vi "STAGE+mono+counter_edit5.vi"() -> ()   [LabVIEW 2017]
panel:
  out "Spectrum 2":waveform(dbl)(graph)
  out "XY Graph":cluster{"Y":dbl[], "Y":dbl[]}[](graph)
  in  "Integrating time, 10^-7 sec":dbl=10000000.0
  out "Timeout 2":bool
  in  "scan from":i32=2600
  in  "scan to":i32=4000
  in  "?":bool
  in  "Exit Labview":bool
  in  "step size":dbl=10.0 min=0.0
  in  "?":bool
  out "Spectrum":waveform(dbl)(graph)
  out "Counts":i32
  in  "value (0)":dbl=-9.0
  out "Current WL Wavelength  2":u16 caption="Current Wavelength"
  out "Grt# 2":u8=1 min=1 max=3 step=1
  out "Blaze (nm)":u32=300
  out "Groove/mm":u32=1200
  in  "?":bool
  in  "Channel B Input":u16(ring)=2 items=["Input 1"=1, "Input 2"=2]
  in  "Trigger mode":u16(ring) items=["10 MHz"=0, "Input 2"=2, "Input T"=3]
  out "Current WL Wavelength":u16 caption="Current Wavelength"
  in  "Integrating time, 10^-7 sec":dbl=10000000.0
  in  "gate A mode (CW:0)":i16(slide) scale=0.0..2.0 scale format="%.2f"
  in  "Channel A Input":u16(ring)=1 items=["10 MHz", "Input 1"]
  in  "Time between measurements\n at one point (s)/Dwell Time":dbl=0.002 min=0.002 max=60.0 step=0.001
  in  "Number of Measurements\n to take at one point/ Number of Periods":u16=1 min=1 max=2000 step=1
  in  "Count Mode":u16(ring) items=["A,B for Preset T", "A-B for Preset T", "A+B for Preset T", "A for Preset B"]
  in  "GPIB address":string="23"
  out "Timeout":bool
  out "Serial":u32=12345
  out "Grt#":u8=1 min=1 max=3 step=1
  out "Blaze (nm)":u32=300
  out "Groove/mm":u32=1200
  out "time delay":u32=450000 min=1
  out "Mono port":T1(ring)
  in  "Get position":bool
  out "Position status":dbl format="%.3f"
  in  "Target position":dbl format="%.3f"
  in  "Move":bool
  in  "Motor OFF":bool
  in  "Motor ON":bool
  in  "Step Size [um]":i32=10
  in  "Axis":i32=1
  in  "Rep Rate [Hz]":dbl=500.0
  out "Shots":dbl
  in  "Averaging Time [s]":dbl=0.1
  out "Current Point":i32
  out "Slide":i32(slide) scale=0.0..100.0
  out "Current Position [mm]":dbl
  in  "Axis initial position [mm]":dbl
  out "Axis final Position [mm]":dbl
  in  "Data Points (100 default)":i32=100
  in  "Collect Data!":bool
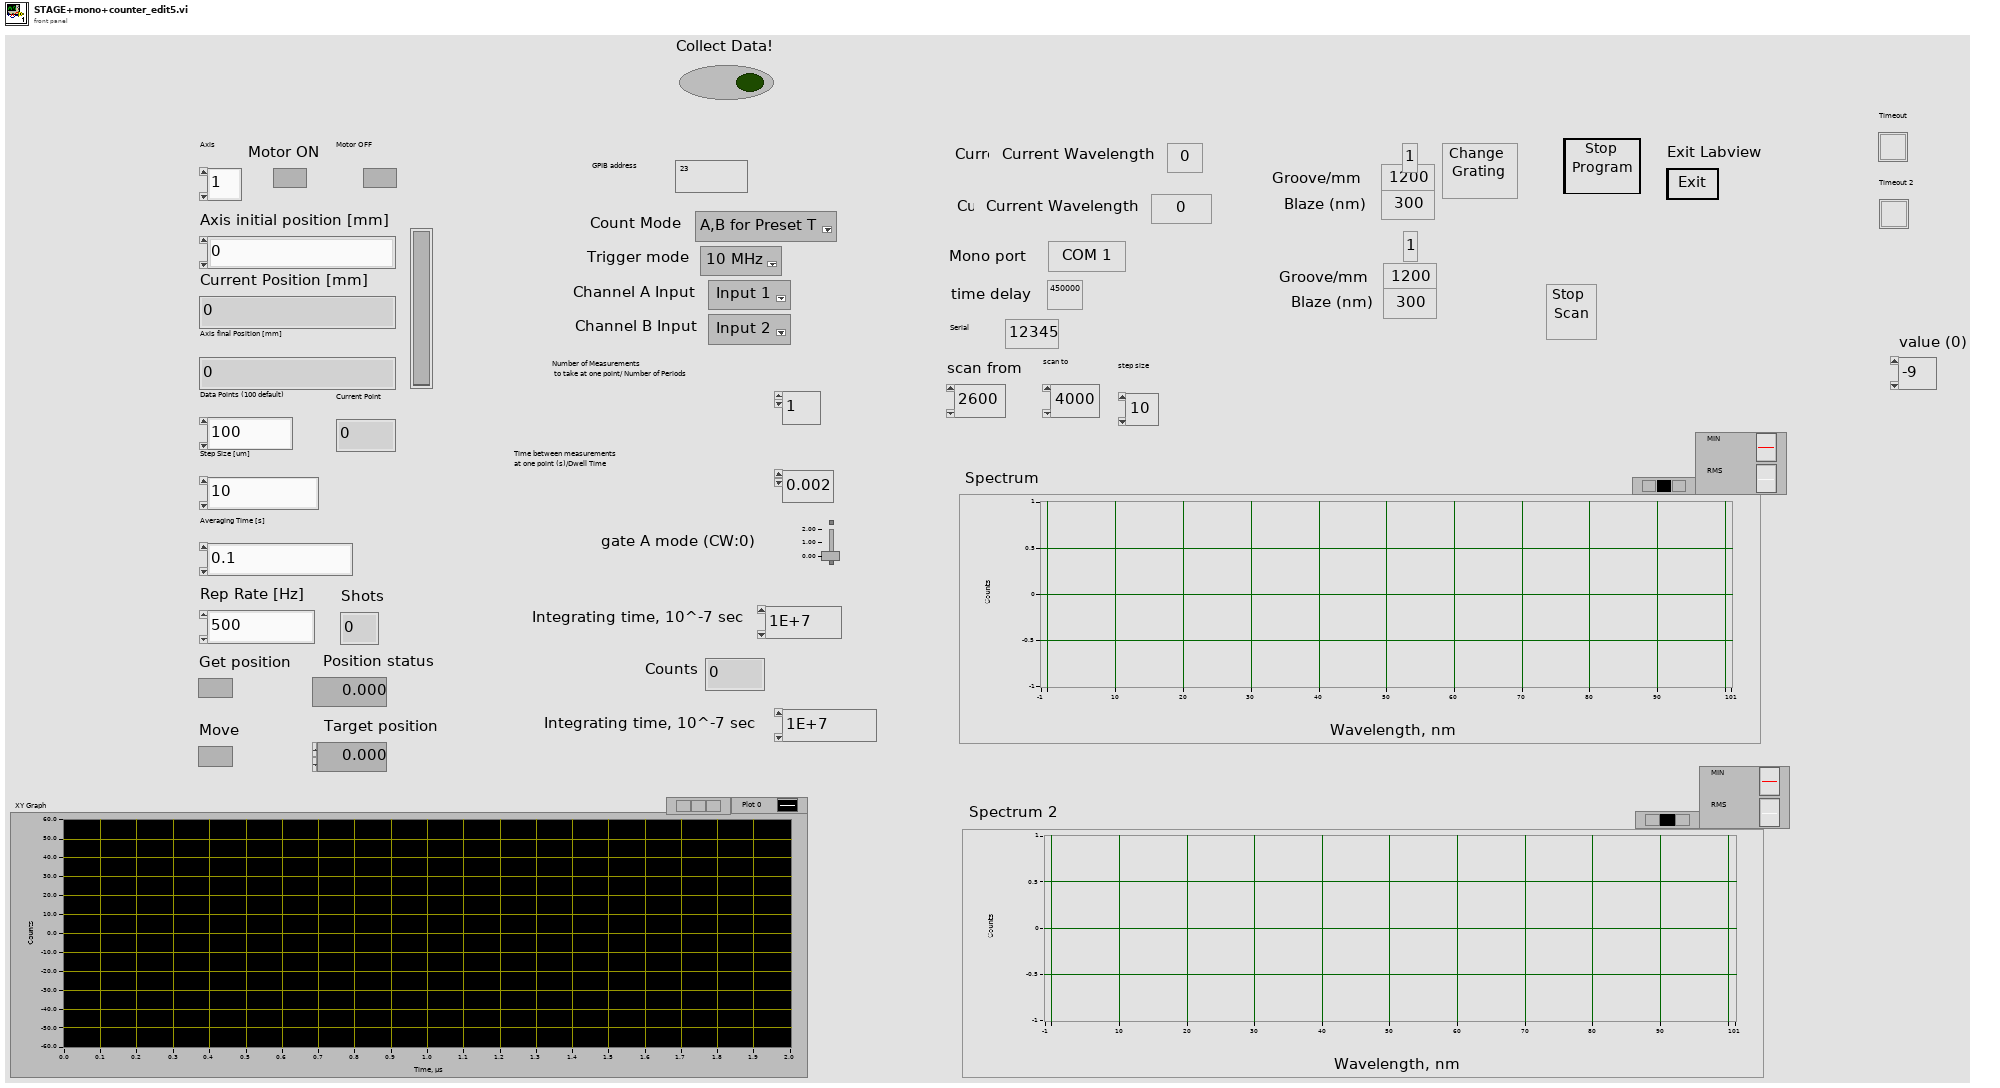
[diagram p1: front panel]
types:
  T1 = enum8{"COM 1", "COM 2", "COM 3", "COM 4", "COM 5", "COM 6", "COM 7", "COM 8", "COM 9"}
  T2 = cluster{"input XON/XOFF":bool, "input HW Handshake":bool, "input alt HW HShk":bool, "output XON/XOFF":bool, "output HW Handshake":bool, "output alt HW HShk":bool, "XOFF byte":u8, "XON byte":u8, "parity error byte":u16}
  T3 = enum16{"no parity", "odd parity", "even parity", "mark parity", "space parity"}
  T4 = cluster{"Y[0]":dbl, "Y[1]":dbl, "Y[2]":dbl, "Y[3]":dbl, "Y[4]":dbl, "Y[5]":dbl, "Y[6]":dbl, "Y[7]":dbl, "Y[8]":dbl}
  T5 = typedef "NI_Matrix.lvlib/RealMatrix.ctl" = dbl[][]
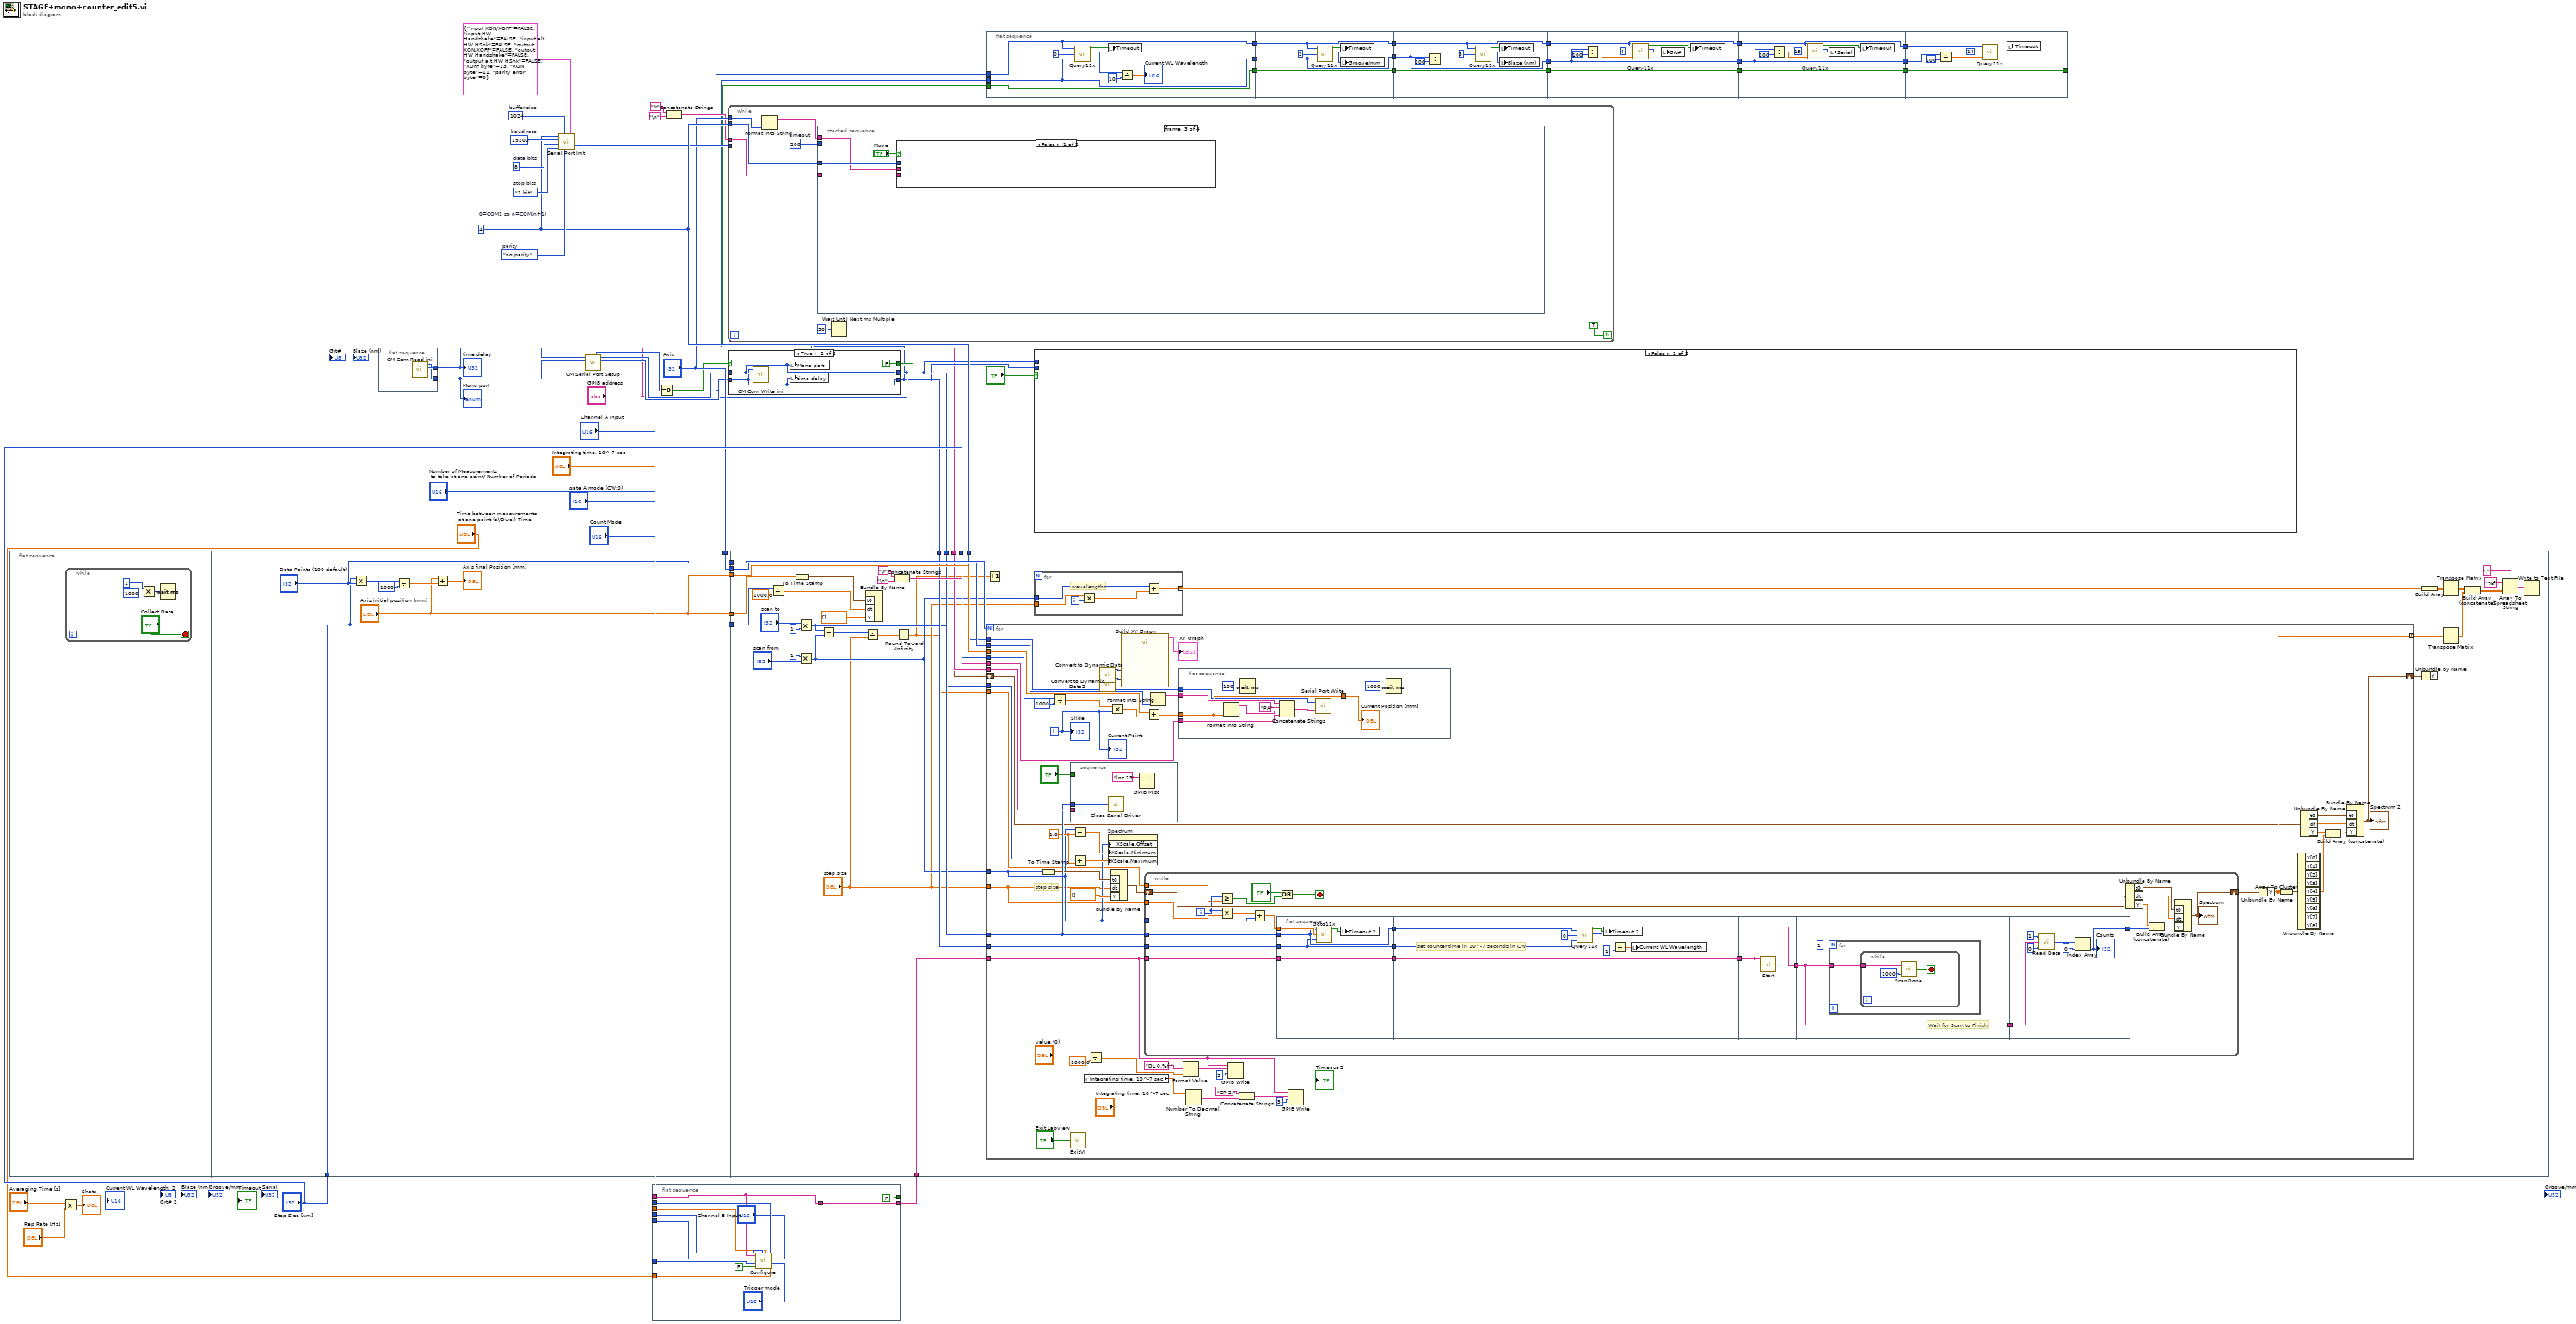
[diagram p0: block diagram]
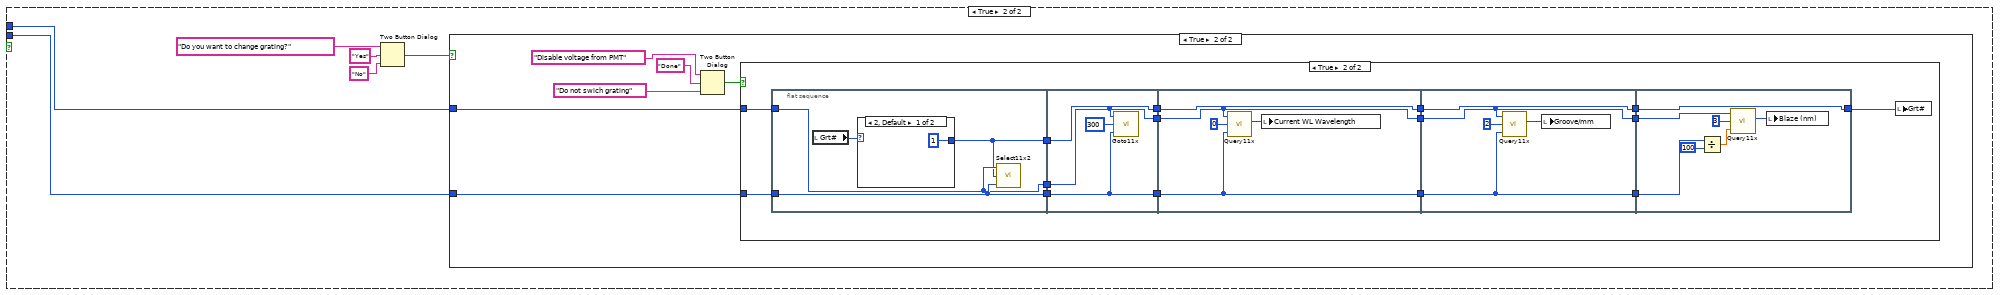
[diagram p2: hidden frame]
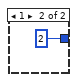
[diagram p5: hidden frame]
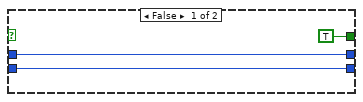
[diagram p6: hidden frame]
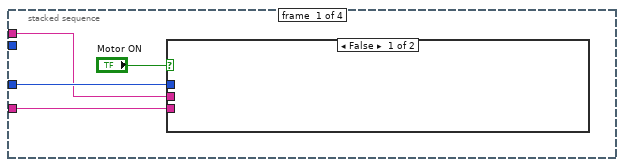
[diagram p7: hidden frame]
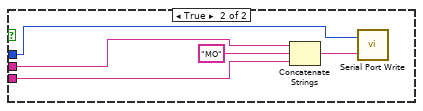
[diagram p8: hidden frame]
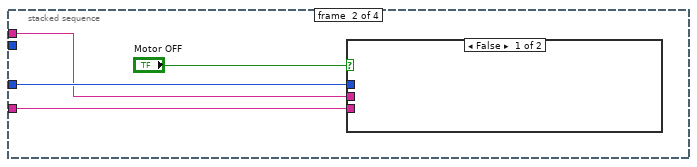
[diagram p9: hidden frame]
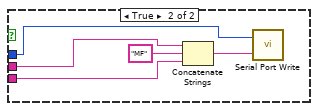
[diagram p10: hidden frame]
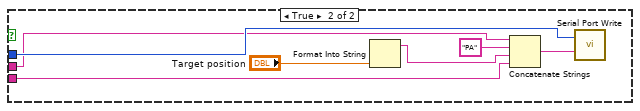
[diagram p11: hidden frame]
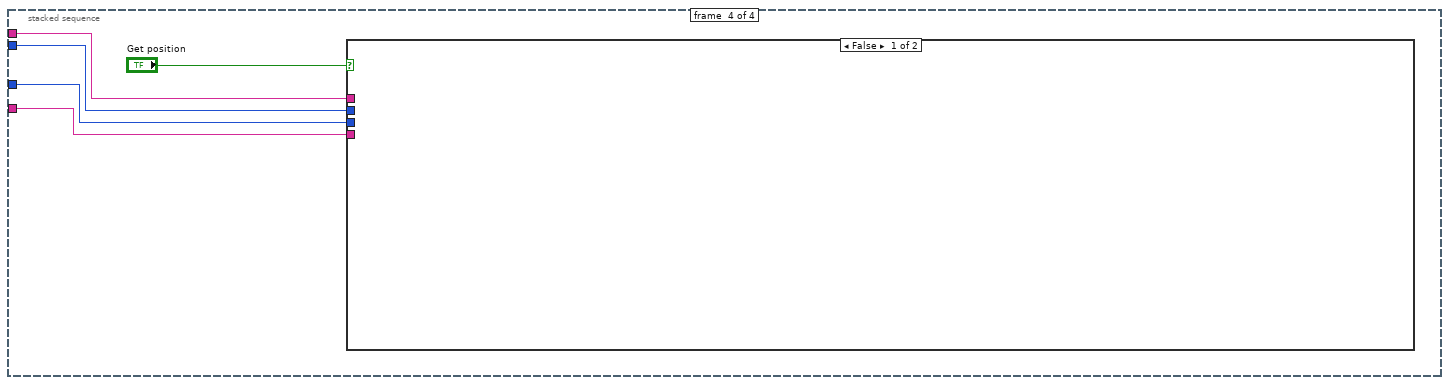
[diagram p12: hidden frame]
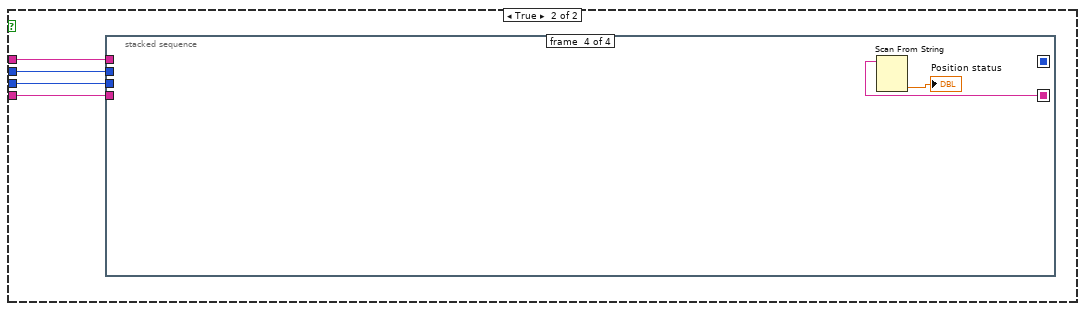
[diagram p13: hidden frame]
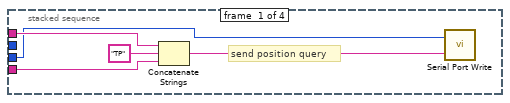
[diagram p14: hidden frame]
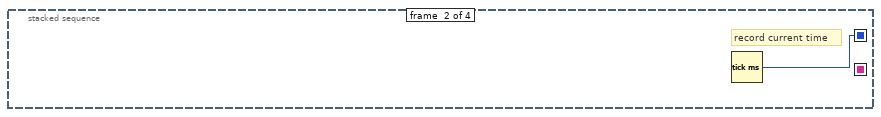
[diagram p15: hidden frame]
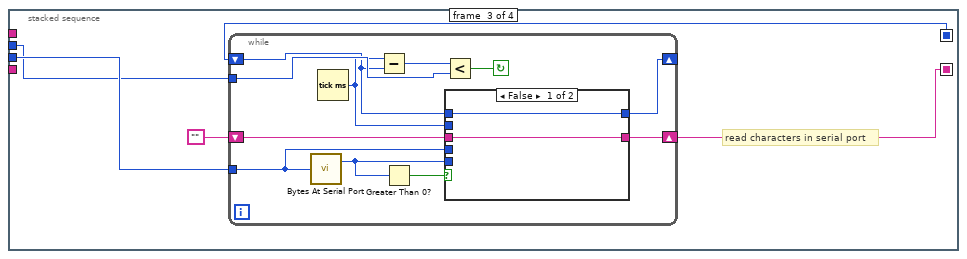
[diagram p16: hidden frame]
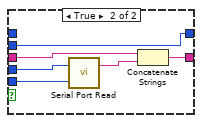
[diagram p17: hidden frame]
diagram:
  w45 = u32 19200  # baud rate
  w44 = u16 8  # data bits
  w43 = enum16{"1 bit", "1.5 bits", "2 bits"}."1 bit"  # stop bits
  w48 = T3."no parity"  # parity
  w42 = 4  # 0=COM1 so n=COM(n+1)
  w47 = u16 1024  # buffer size
  n1 = flat-sequence {
    tunnel: ["Data Points (100 default)"] -> w55
    tunnel: "Axis" -> [w67]
    tunnel: ["Axis initial position [mm]"] -> w54
    tunnel: "Step Size [um]" -> [w60]
    tunnel: [w67] -> w53
    tunnel: ["Axis initial position [mm]"] -> w2
    tunnel: [w60] -> w1
    tunnel: w55 -> [w107]
    tunnel: w54 -> [w106]
    tunnel: "Step Size [um]" -> [w105]
    tunnel: w53 -> [w104]
    tunnel: w42 -> [w100]
    tunnel: w6 -> [w99]
    tunnel: w5 -> [w98]
    tunnel: w4 -> [w97]
    tunnel: "GPIB address" -> [w96]
    tunnel: w2 -> [w75]
    tunnel: w1 -> [w74]
    frame #0 {
      n2 = while {
        stop <- "Collect Data!" stop-if-true
        n3 = Multiply(x=1, y=1000) -> (x*y=w59:i32)
        n4 = Wait (ms)(milliseconds to wait=w59) -> ()  [unwired: 1 out]
      }
    }
    frame #1 {
      n5 = Multiply(x=w60, y="Data Points (100 default)") -> (x*y=w64:i32)
      n6 = Divide(x=w64, y=1000) -> (x/y=w63:dbl)
      n7 = Add(x="Axis initial position [mm]", y=w63) -> (x+y=→"Axis final Position [mm]":dbl)
    }
    frame #2 {
      n8 = Divide(x=w74, y=1000.0) -> (x/y=w72:dbl)
      n9 = To Time Stamp(1:w75) -> (0:w73:timestamp)
      n10 = Multiply(x="scan to", y=1) -> (x*y=w88:i32)
      n11 = Multiply(x=1, y="scan from") -> (x*y=w91:i32)
      n12 = Subtract(x=w88, y=w91) -> (x-y=w86:i32)
      n13 = Divide(x=w86, y="step size") -> (x/y=w85:dbl)
      n14 = Bundle By Name("t0"=w73, "dt"=w72, "Y"=dbl[] []) -> (w69:waveform(dbl))  [unwired: 1 in]
      n15 = Concatenate Strings("\r", "\n") -> (w101:string)
      n16 = Round Toward -Infinity(1:w85) -> (0:w84:dbl)
      n17 = for {
        N: w107 -> [_]
        tunnel: w106 -> [w164]
        tunnel: w105 -> [w160]
        tunnel: w104 -> [w157]
        tunnel: w101 -> [w154]
        tunnel: w100 -> [w155]
        tunnel: w99 -> [w152]
        tunnel: w98 -> [w149]
        tunnel: w97 -> [w151]
        tunnel: w96 -> [w150]
        tunnel: [w121] -> w79 mode=indexing
        tunnel: w91 -> [w130]
        tunnel: w88 -> [w129]
        tunnel: "step size" -> [w128]
        tunnel: w84 -> [w127]
        shift-right: [w113] -> w68
        shift-left: w69 -> [w117]
        i -> [w126]
        w146 = 1.0 ("x")
        # "step size"
        n18 = To Time Stamp(1:w130) -> (0:w142:timestamp)
        n19 = Divide(x=w160, y=1000) -> (x/y=w159:dbl)
        n20 = stacked-sequence {
          tunnel: "?" -> [_]
          tunnel: w149 -> [w217]
          tunnel: w150 -> [_]
          frame #0 {
            n21 = call <vilib>:"Close Serial Driver.vi"("port number"=w217) -> ()  [unwired: 1 out]
            n22 = GPIB Misc(0:"loc 23" ("command string")) -> ()  [unwired: 1 in, 3 out]
          }
        }
        n23 = call "ExitVI.vi"("Exit Labview"="Exit Labview") -> ()
        n24 = Subtract(x=w130, y=w146) -> (x-y=w145:dbl)
        n25 = Add(x=w129, y=w146) -> (x+y=w147:dbl)
        n26 = local read "Integrating time, 10^-7 sec"() -> (w144:dbl)
        n27 = Divide(x="value (0)", y=1000.0) -> (x/y=w131:dbl)
        n28 = call "Convert to Dynamic Data"() -> ("Dynamic Data Type"=w123:dynamicdata)  [unwired: 4 in]
        n29 = call "Convert to Dynamic Data2"() -> ("Dynamic Data Type"=w124:dynamicdata)  [unwired: 4 in]
        n30 = property on="Spectrum" class="WFGraph (strict)"("XScale.Offset"=w130, "XScale.Minimum"=w145, "XScale.Maximum"=w147) -> ()  [unwired: 2 in, 2 out]
        n31 = Multiply(x=w159, y=w126) -> (x*y=w163:dbl)
        n32 = Bundle By Name("t0"=w142, "dt"=w128, "Y"=dbl[] []) -> (w141:waveform(dbl))  [unwired: 1 in]
        n33 = call "Build XY Graph"("Y Input"=w124, "X Input"=w123) -> ("XY Graph"=→"XY Graph":cluster{"Y":dbl[], "Y":dbl[]}[])  [unwired: 3 in, 6 out]
        n34 = while {
          tunnel: w149 -> [w188]
          tunnel: w151 -> [w187]
          shift-right: [w177] -> w136
          shift-left: w141 -> [w185]
          tunnel: w152 -> [w176]
          tunnel: w130 -> [w167]
          tunnel: w128 -> [w166]
          tunnel: w127 -> [w165]
          i -> [w182]
          stop <- w186 stop-if-true
          n35 = Greater Or Equal?(x=w182, y=w165) -> (x >= y?=w178:bool)
          n36 = Multiply(x=w182, y=w166) -> (x*y=w189:dbl)
          n37 = Add(x=w189, y=w167) -> (x+y=w168:dbl)
          n38 = flat-sequence {
            tunnel: w168 -> [w194]
            tunnel: w188 -> [w193]
            tunnel: [w193] -> w174
            tunnel: w187 -> [w192]
            tunnel: [w192] -> w173
            tunnel: w176 -> [w190]
            tunnel: [w190] -> w172
            tunnel: w174 -> [w201]
            tunnel: w173 -> [w200]
            tunnel: w172 -> [w198]
            tunnel: [w198] -> w171
            tunnel: w171 -> [w203]
            tunnel: [w203] -> w170
            tunnel: w170 -> [w204]
            tunnel: [w204] -> w169
            tunnel: w169 -> [w211]
            tunnel: [w210] -> w175
            frame #0 {
              n39 = call "Goto11x.vi"("time delay"=w192, "WAVELENGTH"=w194, "port number"=w193) -> ("timeout"=w191:bool)  [unwired: 2 out]
              n40 = local write "Timeout 2"(w191) -> ()
            }
            frame #1 {
              # "set counter time in 10^-7 seconds in CW"
              n41 = call "Query11x.vi"("port number"=w201, "QUERY"=0, "time delay"=w200) -> ("timeout"=w199:bool, "STATUS MESSAGE"=w197:u16)  [unwired: 2 out]
              n42 = local write "Timeout 2"(w199) -> ()
              n43 = Divide(x=w197, y=1) -> (x/y=w196:dbl)
              n44 = local write "Current WL Wavelength"(w196) -> ()
            }
            frame #2 {
              n45 = call "Start.vi"("GPIB Address"=w203) -> ()  [unwired: 9 in]
            }
            frame #3 {
              # "Wait for Scan to Finish"
              n46 = for {
                N: 1 -> [_]
                tunnel: w204 -> [w206]
                n47 = while {
                  tunnel: w206 -> [w207]
                  stop <- w209 stop-if-true
                  n48 = call "ScanDone.vi"("Wait (ms)"=1000, "GPIB Address"=w207) -> ("Scan Finished?"=w209:bool)
                }
              }
            }
            frame #4 {
              n49 = call "Read Data.vi"("Channel Number"=0, "GPIB Address"=w211, "Number of Datapoints"=1) -> ("Data"=w212:i32[])
              n50 = Index Array(array=w212, index=0) -> (element=w210:i32)
              "Counts" <- w210
            }
          }
          n51 = Or(x="?", y=w178) -> (x .or. y?=w186:bool)
          n52 = Unbundle By Name(w185) -> ("t0"=w183:timestamp, "dt"=w184:dbl, "Y"=w181:dbl[])
          n53 = Build Array (concatenate)(w181, w175) -> (w180:dbl[])
          n54 = Bundle By Name("t0"=w183, "dt"=w184, "Y"=w180) -> (w177:waveform(dbl))  [unwired: 1 in]
          "Spectrum" <- w177
        }
        n55 = Add(x=w164, y=w163) -> (x+y=w162:dbl)
        n56 = Format Into String(w157) -> (resulting string=w156:string)  [unwired: 3 in, 1 out]
        n57 = flat-sequence {
          tunnel: w162 -> [w220]
          tunnel: [w220] -> w158
          tunnel: w154 -> [w222]
          tunnel: w156 -> [w221]
          tunnel: w155 -> [w218]
          tunnel: w158 -> [w226]
          frame #0 {
            n58 = Format Into String(w220) -> (resulting string=w219:string)  [unwired: 3 in, 1 out]
            n59 = Wait (ms)(milliseconds to wait=u32 100) -> ()  [unwired: 1 out]
            n60 = Concatenate Strings(w221, "PA" ("Substring"), w219, w222) -> (w224:string)
            n61 = call <vilib>:"Serial Port Write.vi"("string to write"=w224, "port number"=w218) -> ()  [unwired: 1 out]
          }
          frame #1 {
            n62 = Wait (ms)(milliseconds to wait=u32 1000) -> ()  [unwired: 1 out]
            "Current Position [mm]" <- w226
          }
        }
        n63 = Format Value(format string="DL 0,%f;", value (0)=w131) -> (output string=w134:string)  [unwired: 1 in]
        n64 = Number To Decimal String(number=w144) -> (decimal integer string=w139:string)  [unwired: 1 in]
        n65 = GPIB Write(0:w152, 1:w134, 2:i16 5 ("mode (0)")) -> ()  [unwired: 2 in, 2 out]
        n66 = Concatenate Strings("CP 2,", w139) -> (w137:string)
        n67 = GPIB Write(0:w152, 1:w137, 2:i16 5 ("mode (0)")) -> ()  [unwired: 2 in, 2 out]
        n68 = Unbundle By Name(w136) -> ("Y"=w121:dbl[])
        n69 = Array To Cluster(array=w121) -> (cluster=w120:T4)
        n70 = Unbundle By Name(w120) -> ("Y[4]"=w116:dbl)  [unwired: 8 out]
        n71 = Unbundle By Name(w117) -> ("t0"=w119:timestamp, "dt"=w118:dbl, "Y"=w115:dbl[])
        n72 = Build Array (concatenate)(w115, w116) -> (w114:dbl[])
        n73 = Bundle By Name("t0"=w119, "dt"=w118, "Y"=w114) -> (w113:waveform(dbl))  [unwired: 1 in]
        "Spectrum 2" <- w113
        "Current Point" <- w126
        "Slide" <- w126
      }
      n74 = Increment(x=w84) -> (x+1=w83:dbl)
      n75 = for {
        N: w83 -> [_]
        tunnel: "step size" -> [w112]
        tunnel: w91 -> [w110]
        tunnel: [w108] -> w81 mode=indexing
        i -> [w111]
        # "wavelengths"
        n76 = Multiply(x=w112, y=w111) -> (x*y=w109:dbl)
        n77 = Add(x=w110, y=w109) -> (x+y=w108:dbl)
      }
      n78 = Build Array(w81) -> (w80:dbl[][])
      n79 = Unbundle By Name(w68) -> ()  [unwired: 1 out]
      n80 = Transpose Matrix(1:w80) -> (0:w78:dbl[][])
      n81 = Transpose Matrix(1:w79) -> (0:w77:dbl[][])
      n82 = Build Array (concatenate)(w78, w77) -> (w76:T5)
      n83 = Array To Spreadsheet String(delimiter (Tab)=",", array=w76, 3:"%f" ("format string")) -> (spreadsheet string=w82:string)
      n84 = Write to Text File(text=w82) -> ()  [unwired: 3 in, 3 out]
    }
  }
  n85 = Multiply(x="Averaging Time [s]", y="Rep Rate [Hz]") -> (x*y=→"Shots":dbl)
  n86 = flat-sequence {
    tunnel: [w229] -> w20
    tunnel: [w228] -> w19
    frame #0 {
      n87 = call "CM Com Read ini.vi"() -> ("Mono port"=w228:T1, "time delay1"=w229:u32)  [unwired: 7 in]
    }
  }
  n88 = call <vilib>:"Serial Port Init.vi"("flow control etc."=T2 {"input XON/XOFF"=FALSE, "input HW Handshake"=FALSE, "input alt HW HShk"=FALSE, "output XON/XOFF"=FALSE, "output HW Handshake"=FALSE, "output alt HW HShk"=FALSE, "XOFF byte"=13, "XON byte"=11, "parity error byte"=0}, "parity"=w48, "buffer size"=w47, "stop bits"=w43, "data bits"=w44, "baud rate"=w45, "port number"=w42) -> ("error code"=w41:i32)
  n89 = call "CM Serial Port Setup.vi"("COM port"=w19, "time delay"=w20) -> ("time delay1"=w15:u32, "DK port Out"=w16:T1, "error code"=w18:i32)  [unwired: 7 in]
  n90 = flat-sequence {
    tunnel: "GPIB address" -> [w237]
    tunnel: [w237] -> w21
    tunnel: "Count Mode" -> [w238]
    tunnel: "Number of Measurements\n to take at one point/ Number of Periods" -> [w235]
    tunnel: "Time between measurements\n at one point (s)/Dwell Time" -> [w234]
    tunnel: "Channel A Input" -> [w239]
    tunnel: "gate A mode (CW:0)" -> [w231]
    tunnel: "Integrating time, 10^-7 sec" -> [w230]
    tunnel: w21 -> [w240]
    tunnel: [w240] -> w6
    tunnel: [FALSE] -> _
    frame #0 {
      n91 = call "Configure.vi"("Dwell Time (s)"=w234, "Channel T Input"="Trigger mode", "Channel B Input"="Channel B Input", "Channel A Input"=w239, "Integrating time, 10^-7 sec"=w230, "gate mode (CW:0)"=w231, "Scan End Mode"=FALSE, "Number of Periods"=w235, "Count Mode"=w238, "GPIB Address"=w237) -> ()
    }
    frame #1 {
    }
  }
  n92 = Equal To 0?(x=w18) -> (x = 0?=w17:bool)
  n93 = Concatenate Strings("\r", "\n") -> (w37:string)
  n94 = while {
    tunnel: w42 -> [w244]
    tunnel: w37 -> [w245]
    tunnel: w41 -> [_]
    tunnel: "Axis" -> [w242]
    stop <- TRUE continue-if-true
    w243 = u32 200  # timeout
    n95 = Format Into String(w242) -> (resulting string=w246:string)  [unwired: 3 in, 1 out]
    n96 = stacked-sequence {
      tunnel: w246 -> [w250 w260 w269 w281]
      tunnel: w245 -> [w249 w259 w268 w278]
      tunnel: w244 -> [w251 w261 w270 w280]
      tunnel: w243 -> [_ _ _ w279]
      frame #0 {
        n97 = case shown="False" "Motor ON" {
          tunnel: w251 -> [_ w257]
          tunnel: w250 -> [_ w254]
          tunnel: w249 -> [_ w253]
          frame False {
          }
          frame True {
            n98 = Concatenate Strings(w254, "MO" ("Substring"), w253) -> (w255:string)
            n99 = call <vilib>:"Serial Port Write.vi"("string to write"=w255, "port number"=w257) -> ()  [unwired: 1 out]
          }
        }
      }
      frame #1 {
        n100 = case shown="False" "Motor OFF" {
          tunnel: w261 -> [_ w266]
          tunnel: w260 -> [_ w263]
          tunnel: w259 -> [_ w262]
          frame False {
          }
          frame True {
            n101 = Concatenate Strings(w263, "MF" ("Substring"), w262) -> (w264:string)
            n102 = call <vilib>:"Serial Port Write.vi"("string to write"=w264, "port number"=w266) -> ()  [unwired: 1 out]
          }
        }
      }
      frame #2 {
        n103 = case shown="False" "Move" {
          tunnel: w270 -> [_ w277]
          tunnel: w269 -> [_ w274]
          tunnel: w268 -> [_ w273]
          frame False {
          }
          frame True {
            n104 = Format Into String("Target position") -> (resulting string=w271:string)  [unwired: 3 in, 1 out]
            n105 = Concatenate Strings(w274, "PA" ("Substring"), w271, w273) -> (w275:string)
            n106 = call <vilib>:"Serial Port Write.vi"("string to write"=w275, "port number"=w277) -> ()  [unwired: 1 out]
          }
        }
      }
      frame #3 {
        n107 = case shown="False" "Get position" {
          tunnel: w281 -> [_ w286]
          tunnel: w280 -> [_ w285]
          tunnel: w279 -> [_ w284]
          tunnel: w278 -> [_ w283]
          frame False {
          }
          frame True {
            n108 = stacked-sequence {
              seq-local: [_ w292 _ _] -> [_ _ w294 _]
              seq-local: [_ _ w293 _] -> [_ _ _ w318]
              tunnel: w286 -> [w289 _ _ _]
              tunnel: w285 -> [w288 _ w297 _]
              tunnel: w284 -> [_ _ w295 _]
              tunnel: w283 -> [w287 _ _ _]
              frame #0 {
                # "send position query"
                n109 = Concatenate Strings(w289, "TP" ("Substring"), w287) -> (w290:string)
                n110 = call <vilib>:"Serial Port Write.vi"("string to write"=w290, "port number"=w288) -> ()  [unwired: 1 out]
              }
              frame #1 {
                # "record current time"
                n111 = Tick Count (ms)() -> (millisecond timer value=w292:u32)
              }
              frame #2 {
                # "read characters in serial port"
                n112 = while {
                  shift-left: w294 -> [w298]
                  shift-right: [w299] -> _
                  tunnel: w295 -> [w302]
                  shift-left: "" -> [w305]
                  shift-right: [w304] -> w293
                  tunnel: w297 -> [w306]
                  stop <- w301 continue-if-true
                  n113 = call <vilib>:"Bytes At Serial Port.vi"("port number"=w306) -> ("byte count"=w307:u32)  [unwired: 1 out]
                  n114 = Tick Count (ms)() -> (millisecond timer value=w300:u32)
                  n115 = Subtract(x=w300, y=w298) -> (x-y=w303:u32)
                  n116 = Greater Than 0?(x=w307) -> (x > 0?=w308:bool)
                  n117 = Less?(x=w303, y=w302) -> (x < y?=w301:bool)
                  n118 = case shown="False" w308 {
                    tunnel: w307 -> [_ w316]
                    tunnel: w306 -> [_ w315]
                    tunnel: w305 -> [w310 w313]
                    tunnel: [w310 w312] -> w304
                    tunnel: [w309 w311] -> w299
                    tunnel: w300 -> [_ w311]
                    tunnel: w298 -> [w309 _]
                    frame False {
                    }
                    frame True {
                      n119 = call <vilib>:"Serial Port Read.vi"("requested byte count"=w316, "port number"=w315) -> ("string read"=w314:string)  [unwired: 1 out]
                      n120 = Concatenate Strings(w313, w314) -> (w312:string)
                    }
                  }
                }
              }
              frame #3 {
                n121 = Scan From String(input string=w318) -> (output 1=→"Position status":dbl)  [unwired: 4 in, 3 out]
              }
            }
          }
        }
      }
    }
    n122 = Wait Until Next ms Multiple(millisecond multiple=u32 50) -> ()  [unwired: 1 out]
  }
  n123 = case shown="True" w17 {
    tunnel: w16 -> [w321 w324]
    tunnel: w15 -> [w320 w323]
    tunnel: [w321 w324] -> w5
    tunnel: [w320 w323] -> w4
    tunnel: [TRUE FALSE] -> w14
    frame False {
    }
    frame True {
      n124 = call "CM Com Write ini.vi"("time delay1"=w324, "Mono port"=w323) -> ()  [unwired: 7 in]
      n125 = local write "Mono port"(w324) -> ()
      n126 = local write "time delay"(w323) -> ()
    }
  }
  n127 = flat-sequence {
    tunnel: w4 -> [w330]
    tunnel: [w330] -> w36
    tunnel: w5 -> [w332]
    tunnel: [w332] -> w35
    tunnel: w14 -> [w328]
    tunnel: [w328] -> w34
    tunnel: w36 -> [w335]
    tunnel: [w335] -> w33
    tunnel: w35 -> [w337]
    tunnel: [w337] -> w32
    tunnel: w34 -> [w333]
    tunnel: [w333] -> w31
    tunnel: w33 -> [w345]
    tunnel: [w345] -> w30
    tunnel: w32 -> [w342]
    tunnel: [w342] -> w29
    tunnel: w31 -> [w339]
    tunnel: [w339] -> w28
    tunnel: w30 -> [w353]
    tunnel: [w353] -> w27
    tunnel: w29 -> [w350]
    tunnel: [w350] -> w26
    tunnel: w28 -> [w347]
    tunnel: [w347] -> w25
    tunnel: w27 -> [w361]
    tunnel: [w361] -> w24
    tunnel: w26 -> [w358]
    tunnel: [w358] -> w23
    tunnel: w25 -> [w355]
    tunnel: [w355] -> w22
    tunnel: w24 -> [w368]
    tunnel: w23 -> [w365]
    tunnel: [w363] -> _
    tunnel: w22 -> [w363]
    frame #0 {
      n128 = call "Query11x.vi"("port number"=w332, "QUERY"=u16 0, "time delay"=w330) -> ("timeout"=w329:bool, "STATUS MESSAGE"=w327:u16)  [unwired: 2 out]
      n129 = local write "Timeout"(w329) -> ()
      n130 = Divide(x=w327, y=10 ("Numeric")) -> (x/y=→"Current WL Wavelength":dbl)
    }
    frame #1 {
      n131 = call "Query11x.vi"("port number"=w337, "QUERY"=u16 2, "time delay"=w335) -> ("timeout"=w334:bool, "STATUS MESSAGE"=w336:u16)  [unwired: 2 out]
      n132 = local write "Timeout"(w334) -> ()
      n133 = local write "Groove/mm"(w336) -> ()
    }
    frame #2 {
      n134 = Divide(x=w345, y=i16 100 ("device (1)")) -> (x/y=w343:dbl)
      n135 = call "Query11x.vi"("port number"=w342, "QUERY"=u16 3, "time delay"=w343) -> ("timeout"=w340:bool, "STATUS MESSAGE"=w341:u16)  [unwired: 2 out]
      n136 = local write "Timeout"(w340) -> ()
      n137 = local write "Blaze (nm)"(w341) -> ()
    }
    frame #3 {
      n138 = Divide(x=w353, y=i16 100 ("device (1)")) -> (x/y=w351:dbl)
      n139 = call "Query11x.vi"("port number"=w350, "QUERY"=u16 4, "time delay"=w351) -> ("timeout"=w348:bool, "STATUS MESSAGE"=w349:u16)  [unwired: 2 out]
      n140 = local write "Grt#"(w349) -> ()
      n141 = local write "Timeout"(w348) -> ()
    }
    frame #4 {
      n142 = Divide(x=w361, y=i16 100 ("device (1)")) -> (x/y=w359:dbl)
      n143 = call "Query11x.vi"("port number"=w358, "QUERY"=u16 19, "time delay"=w359) -> ("timeout"=w356:bool, "STATUS MESSAGE"=w357:u16)  [unwired: 2 out]
      n144 = local write "Serial"(w357) -> ()
      n145 = local write "Timeout"(w356) -> ()
    }
    frame #5 {
      n146 = Divide(x=w368, y=i16 100 ("device (1)")) -> (x/y=w366:dbl)
      n147 = call "Query11x.vi"("port number"=w365, "QUERY"=u16 14, "time delay"=w366) -> ("timeout"=w364:bool)  [unwired: 3 out]
      n148 = local write "Timeout"(w364) -> ()
    }
  }
  n149 = case shown="False" "?" {
    tunnel: w4 -> [_ w371]
    tunnel: w5 -> [_ w370]
    frame False {
    }
    frame True {
      n150 = Two Button Dialog(message="Do you want to change grating?", 1:"No" ("F button name (\"Cancel\")"), 2:"Yes" ("T button name (\"OK\")")) -> (T button?=w372:bool)
      n151 = case shown="True" w372 {
        tunnel: w371 -> [_ w377]
        tunnel: w370 -> [_ w376]
        frame False {
        }
        frame True {
          n152 = Two Button Dialog(message="Disable voltage from PMT", 1:"Do not swich grating" ("F button name (\"Cancel\")"), 2:"Done" ("T button name (\"OK\")")) -> (T button?=w378:bool)
          n153 = case shown="True" w378 {
            tunnel: w377 -> [_ w396]
            tunnel: w376 -> [_ w395]
            frame False {
            }
            frame True {
              n154 = flat-sequence {
                tunnel: w396 -> [w400]
                tunnel: [w400] -> w393
                tunnel: w395 -> [w399]
                tunnel: [w399] -> w392
                tunnel: [w397] -> w391
                tunnel: w393 -> [w404]
                tunnel: [w404] -> w390
                tunnel: w392 -> [w405]
                tunnel: [w405] -> w389
                tunnel: w391 -> [w403]
                tunnel: [w403] -> w388
                tunnel: w390 -> [w411]
                tunnel: [w411] -> w387
                tunnel: w389 -> [w410]
                tunnel: [w410] -> w386
                tunnel: w388 -> [w407]
                tunnel: [w407] -> w385
                tunnel: w387 -> [w414]
                tunnel: [w414] -> w384
                tunnel: w386 -> [w415]
                tunnel: [w415] -> w383
                tunnel: w385 -> [w412]
                tunnel: [w412] -> w382
                tunnel: w384 -> [w419]
                tunnel: w383 -> [w420]
                tunnel: [w417] -> w394
                tunnel: w382 -> [w417]
                frame #0 {
                  n155 = local read "Grt#"() -> (w398:u8)
                  n156 = case shown="2, Default" w398 {
                    tunnel: [1 2] -> w397
                    frame 2, Default {
                    }
                    frame 1 {
                    }
                  }
                  n157 = call "Select11x2.vi"("time delay"=w400, "NEW GRT?"=w397, "port number"=w399) -> ()  [unwired: 3 out]
                }
                frame #1 {
                  n158 = call "Goto11x.vi"("time delay"=w404, "WAVELENGTH"=u16 300, "port number"=w405) -> ()  [unwired: 3 out]
                }
                frame #2 {
                  n159 = call "Query11x.vi"("port number"=w410, "QUERY"=u16 0, "time delay"=w411) -> ("STATUS MESSAGE"=w408:u16)  [unwired: 3 out]
                  n160 = local write "Current WL Wavelength"(w408) -> ()
                }
                frame #3 {
                  n161 = call "Query11x.vi"("port number"=w415, "QUERY"=u16 2, "time delay"=w414) -> ("STATUS MESSAGE"=w413:u16)  [unwired: 3 out]
                  n162 = local write "Groove/mm"(w413) -> ()
                }
                frame #4 {
                  n163 = Divide(x=w419, y=i16 100 ("device (1)")) -> (x/y=w421:dbl)
                  n164 = call "Query11x.vi"("port number"=w420, "QUERY"=u16 3, "time delay"=w421) -> ("STATUS MESSAGE"=w418:u16)  [unwired: 3 out]
                  n165 = local write "Blaze (nm)"(w418) -> ()
                }
              }
              n166 = local write "Grt#"(w394) -> ()
            }
          }
        }
      }
    }
  }
  "Mono port" <- w19
  "time delay" <- w20
